vi "Config Hold Special.vi"(8 "error in":errorcluster, 9 "Trigger Mode (Buffer)":u16(ring)=1 items=["Error", "Buffer"], 11 "VISA resource name":refnum<visa-resource-name>) -> (0 "error out":errorcluster, 3 "VISA resource name out":refnum<visa-resource-name>)   [LabVIEW 2016, in "Andeen-Hagerling 2550.lvlib"]
doc: "This vi determines what happens to external trigger pulses taht arrive when no HOLD 0 command has been executed to receive them. This command allows such pulses to be buffered or to report an error. Execution of this command clears the trigger buffer."
uses:
  Andeen-Hagerling 2550.lvlib
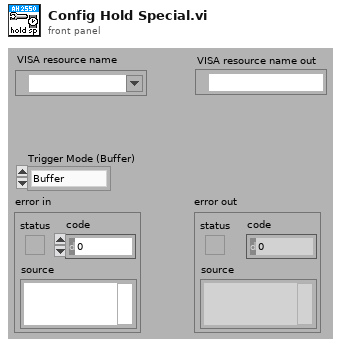
[diagram p1: front panel]
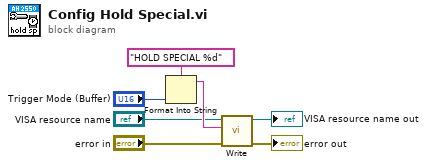
[diagram p0: block diagram]
diagram:
  n1 = Format Into String(format string="HOLD SPECIAL %d", "Trigger Mode (Buffer)") -> (resulting string=w6:string)  [unwired: 2 in, 1 out]
  n2 = call "Write.vi"("error in"="error in", "command"=w6, "VISA resource name"="VISA resource name") -> ("error out"=→"error out":errorcluster, "VISA resource name out"=→"VISA resource name out":refnum<visa-resource-name>)  [unwired: 7 in]
